vi "time_of_move.vi"(1 "导程":dbl=2.0, 2 "转速":i32=2, 3 "移动距离":dbl format="%#_13g") -> (0 "所需时间":i32)   [LabVIEW 2018]
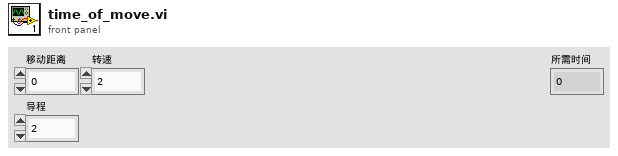
[diagram p1: front panel]
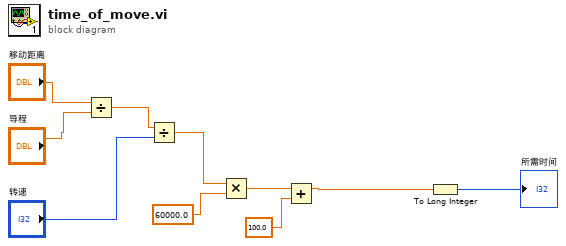
[diagram p0: block diagram]
diagram:
  n1 = Divide(x="移动距离", y="导程") -> (x/y=w8:dbl)
  n2 = Divide(x=w8, y="转速") -> (x/y=w6:dbl)
  n3 = Multiply(x=w6, y=60000.0) -> (x*y=w4:dbl)
  n4 = Add(x=w4, y=100.0) -> (x+y=w3:dbl)
  n5 = To Long Integer(number=w3) -> (32bit integer=→"所需时间":i32)
